vi "Sea-Level SWI Close Device.vi"(8 "error in (no error)":errorcluster, 11 "Handle":i32) -> (0 "error out":errorcluster, 4 "Error Code":T1)   [LabVIEW 2011]
uses:
  TypeDefs/Sea-Level SWI Error Code.ctl
  SeaIo32.dll
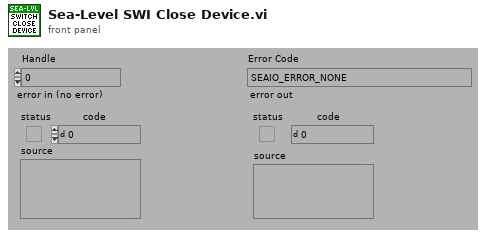
[diagram p1: front panel]
types:
  T1 = typedef "Sea-Level SWI Error Code.ctl" = enum16{"SEAIO_ERROR_NONE", "SEAIO_ERROR_PARAM", "SEAIO_ERROR_NOT_SUPPORTED", "SEAIO_ERROR_PORT_NOT_OPEN", "SEAIO_ERROR_INVALID_NAME", "SEAIO_ERROR_SHARING_VIOLATION", "SEAIO_ERROR_DRIVER_TYPE", "SEAIO_ERROR_BUFFER", "SEAIO_ERROR_INCOMPLETE", "SEAIO_ERROR_GENERAL", "SEAIO_ERROR_IO_PENDING", "SEAIO_ERROR_NO_TXBUFFER", "SEAIO_ERROR_INVALID_DEVICE_REQUEST", "SEAIO_ERROR_INVALID_HANDLE", "SEAIO_ERROR_CANCELED", "SEAIO_ERROR_LAST", "SEAIO_ERROR_NO_MEMORY", "SEAIO_ERROR_BUSY"}
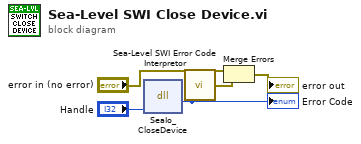
[diagram p0: block diagram]
diagram:
  n1 = dll-call lib="C:/Development/Spartan/www/drivers/SWI/Sea-Level/SeaIo32.dll" fn="SeaIo_CloseDevice"("Handle"="Handle") -> ("Error Code"=w4:i32)  [unwired: 4 in, 2 out]
  "Error Code" <- w4
  n2 = call "Sea-Level SWI Error Code Interpretor.vi"("Error Code"=w4) -> ("error out"=w3:errorcluster)
  n3 = Merge Errors("error in (no error)", w3) -> (→"error out":errorcluster)
